vi "degrees_to_dynamixel_units.vi"(11 "Degree Input":dbl) -> (2 "Dynamixel units/cycle":dbl, 3 "Dynamixel units":dbl)   [LabVIEW 2013]
doc: "This VI takes in degrees and outputs Dynamixel units. The units are different for the MX and AX, which is controlled by the input boolean."
panel:
  in  "MX Motor?":bool
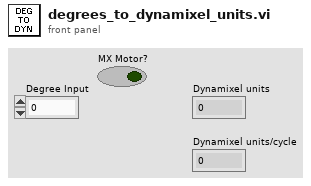
[diagram p1: front panel]
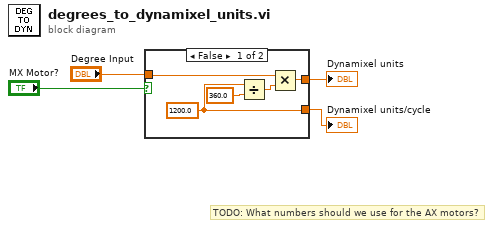
[diagram p0: block diagram]
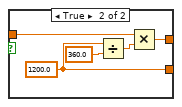
[diagram p2: hidden frame]
diagram:
  # "TODO: What numbers should we use for the AX motors?"
  n1 = case shown="False" "MX Motor?" {
    tunnel: [w5 w14] -> w4
    tunnel: "Degree Input" -> [w6 w13]
    tunnel: [w7 w12] -> w2
    frame False {
      w5 = 1200.0 ("y")
      n2 = Divide(x=w5, y=360.0) -> (x/y=w8:dbl)
      n3 = Multiply(x=w6, y=w8) -> (x*y=w7:dbl)
    }
    frame True {
      w14 = 1200.0 ("y")
      n4 = Divide(x=w14, y=360.0) -> (x/y=w11:dbl)
      n5 = Multiply(x=w13, y=w11) -> (x*y=w12:dbl)
    }
  }
  "Dynamixel units/cycle" <- w4
  "Dynamixel units" <- w2
